vi "Create Message Getter.vi"(7 "RPC Message Name":string, 8 "error in (no error)":errorcluster, 11 "RPC Messages Folder (ProjectItem) in":refnum<vi>) -> (0 "error out":errorcluster, 2 "Message Getter out":refnum<vi>, 3 "RPC Messages Folder (ProjectItem) out":refnum<vi>)   [LabVIEW 2019, in "gRPC Scripting Tools.lvlib"]
uses:
  gRPC Scripting Tools.lvlib
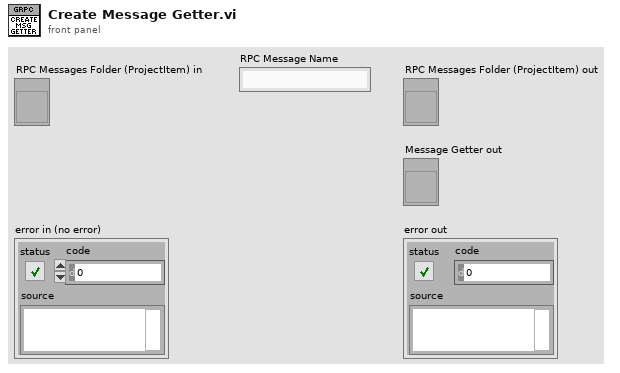
[diagram p1: front panel]
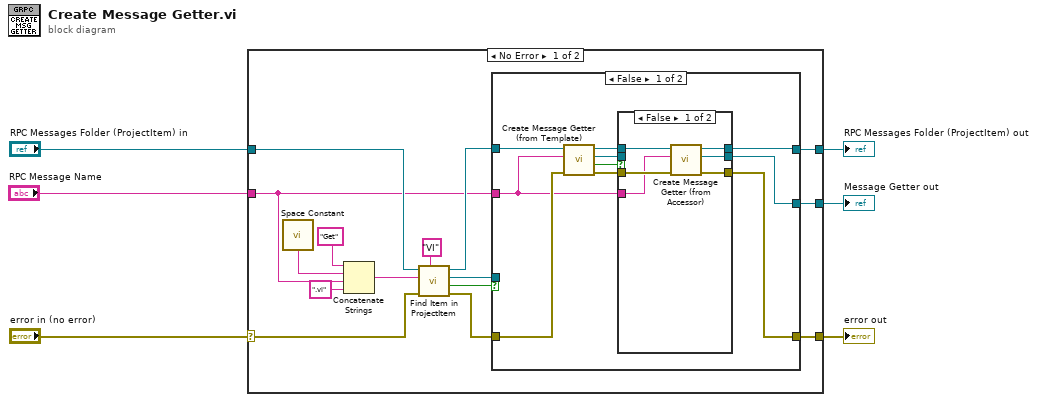
[diagram p0: block diagram]
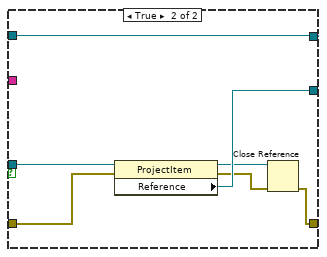
[diagram p3: hidden frame]
diagram:
  n1 = case shown="No Error" "error in (no error)" {
    selector: "error in (no error)" -> [w7 w49]
    tunnel: [w21 _] -> w6
    tunnel: [w20 w48] -> w5
    tunnel: [w19 w49] -> w4
    tunnel: "RPC Messages Folder (ProjectItem) in" -> [w17 w48]
    tunnel: "RPC Message Name" -> [w8 _]
    frame No Error {
      n2 = call <vilib>:"Space Constant.vi"() -> ("String"=w14:string)
      n3 = Concatenate Strings("Get" ("string"), w14, w8, ".vi" ("string")) -> (w12:string)
      n4 = call "Find Item in ProjectItem.vi"("Item Type"="VI", "error in (no error)"=w7, "Name"=w12, "ProjectItem in"=w17) -> ("error out"=w10:errorcluster, "Found ?"=w11:bool, "Item Refnum out"=w9:refnum<vi>, "ProjectItem out"=w16:refnum<vi>)  [unwired: 4 in]
      n5 = case shown="False" w11 {
        tunnel: [w22 w46] -> w21
        tunnel: [w25 w45] -> w20
        tunnel: w10 -> [w31 w42]
        tunnel: [w23 w41] -> w19
        tunnel: w16 -> [w30 w45]
        tunnel: w9 -> [_ w47]
        tunnel: w8 -> [w24 _]
        frame False {
          n6 = call "Create Message Getter (from Template).vi"("error in (no error)"=w31, "RPC Message Name"=w24, "RPC Messages Folder (ProjectItem) in"=w30) -> ("error out"=w28:errorcluster, "Created?"=w29:bool, "Getter VI out"=w26:refnum<vi>, "RPC Messages Folder (ProjectItem) out"=w27:refnum<vi>)  [unwired: 5 in]
          n7 = case shown="False" w29 {
            tunnel: w28 -> [w37 w39]
            tunnel: w27 -> [w36 w40]
            tunnel: w26 -> [_ w38]
            tunnel: [w33 w40] -> w25
            tunnel: [w34 w39] -> w23
            tunnel: [w32 w38] -> w22
            tunnel: w24 -> [w35 _]
            frame False {
              n8 = call "Create Message Getter (from Accessor).vi"("error in (no error)"=w37, "RPC Message Name"=w35, "RPC Messages Folder (ProjectItem) in"=w36) -> ("error out"=w34:errorcluster, "Getter VI out"=w32:refnum<vi>, "RPC Messages Folder (ProjectItem) out"=w33:refnum<vi>)  [unwired: 5 in, 1 out]
            }
            frame True {
            }
          }
        }
        frame True {
          n9 = property class="ProjectItem"(reference=w47, error in=w42) -> (reference out=w43:refnum<vi>, error out=w44:errorcluster, "Reference"=w46:refnum<vi>)
          n10 = Close Reference(reference=w43, error in (no error)=w44) -> (error out=w41:errorcluster)
        }
      }
    }
    frame Error {
    }
  }
  "error out" <- w4
  "Message Getter out" <- w6
  "RPC Messages Folder (ProjectItem) out" <- w5
